vi "serialInitialize_p.vi"(2 "subID2 (nc)":u32, 3 "subID1 (0)":u32, 4 "boardBaseAdd":u32 format="%.0x", 5 "serialBoard":u16(ring) items=["DEVIL", "M17"]) -> (1 "errorCode":cdb format="%.2f")   [LabVIEW 2010]
doc: "Initializes the selected serial communication channel."
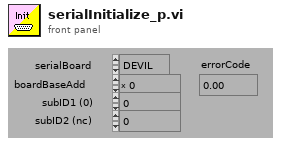
[diagram p1: front panel]
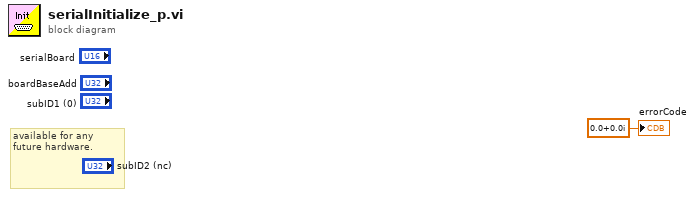
[diagram p0: block diagram]
diagram:
  # "available for any future hardware."
  "errorCode" <- cdb 0.0+0.0i ("errorCode")
